vi "版本号读取.vi"(8 "Error in":errorcluster caption="Error in (no error)", 11 "MB session in":refnum<class "MB_Master.lvclass">) -> (0 "error out":errorcluster, 2 "固件版本号":string, 3 "MB session out":refnum<class "MB_Master.lvclass">)   [LabVIEW 2016, in "斯坦道氨氮V2.lvlib"]
uses:
  <vilib>/Plasmionique/MB Master/MB_Master/MB_Master.lvclass
  <vilib>/Plasmionique/MB Master/MB Master.lvlib
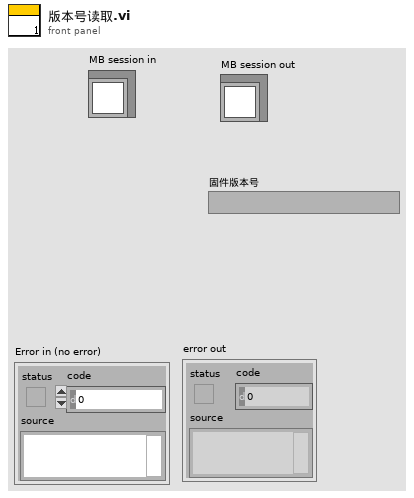
[diagram p1: front panel]
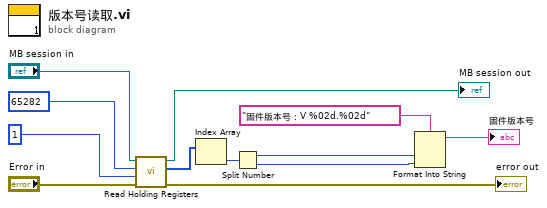
[diagram p0: block diagram]
diagram:
  n1 = call <vilib>:"Read Holding Registers.vi"("error in (no error)"="Error in", "quantity"=u16 1, "starting address"=u16 65282, "MB session in"="MB session in") -> ("error out"=→"error out":errorcluster, "Registers"=w4:u16[], "MB session out"=→"MB session out":refnum<class "MB_Master.lvclass">)  [unwired: 5 in]
  n2 = Index Array(array=w4) -> (element=w6:u16)  [unwired: 1 in]
  n3 = Split Number(x=w6) -> (hi(x)=w2:u8, lo(x)=w1:u8)
  n4 = Format Into String(format string="固件版本号：V %02d.%02d" ("格式字符串"), w2, w1) -> (resulting string=→"固件版本号":string)  [unwired: 2 in, 1 out]
